vi "Path Type Specialization - Single Converter.vi"(11 "error in":errorcluster) -> (4 "type specialization for path":T1(array[cluster]), 15 "error out":errorcluster)   [LabVIEW 2021, in "Converter.lvlib"]
uses:
  Converter.lvlib
  <vilib>/Utility/traverseref.llb/TRef TravTarget.ctl
  <vilib>/Utility/traverseref.llb/VI Scripting - Traverse.lvlib
  Path Functions/Path Functions.lvlib
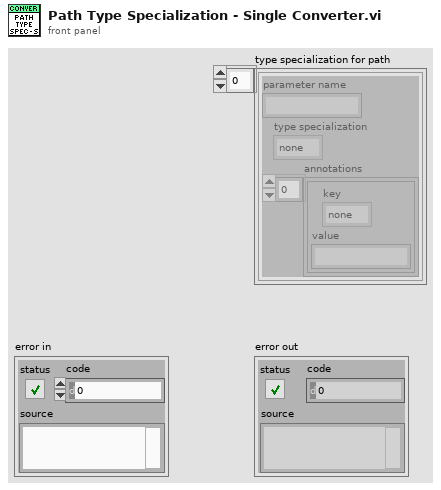
[diagram p1: front panel]
types:
  T1 = cluster{"parameter name":string, "type specialization":enum16{"none", "pin", "path", "enum"}, "annotations":cluster{"key":enum16{"none", "pin.instrument_type", "enum.values"}, "value":string}[]}[]
  T2 = typedef "TRef TravTarget.ctl" = enum16{"FP", "BD", "Other"}
  T3 = cluster{"parameter name":string, "type specialization":enum16{"none", "pin", "path", "enum"}, "annotations":cluster{"key":enum16{"none", "pin.instrument_type", "enum.values"}, "value":string}[]}
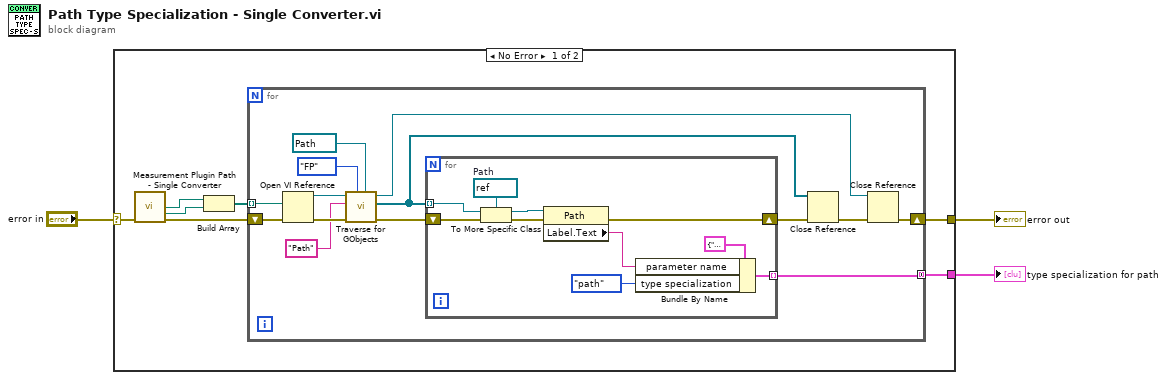
[diagram p0: block diagram]
diagram:
  n1 = case shown="No Error" "error in" {
    selector: "error in" -> [w10 w35]
    tunnel: [w5 w35] -> w2
    tunnel: [w4 _] -> w1
    frame No Error {
      n2 = call "Measurement Plugin Path - Single Converter.vi"("error in"=w10) -> ("result control"=w8:path, "input controls"=w7:path, "error out"=w9:errorcluster)  [unwired: 2 in, 10 out]
      n3 = Build Array(w8, w7) -> (w6:path[])
      n4 = for {
        tunnel: w6 -> [w12] mode=indexing
        shift-right: [w14] -> w5
        shift-left: w9 -> [w23]
        tunnel: [w18] -> w4 mode=concatenating
        n5 = Open VI Reference(vi path=w12, error in (no error)=w23) -> (vi reference=w22:refnum<vi>, error out=w24:errorcluster)  [unwired: 4 in]
        n6 = call <vilib>:"Traverse for GObjects.vi"("Other Refnum"=refnum<vi> refnum, "Traverse Target"=TRef_TravTarget."FP", "error in (no error)"=w24, "Class Name"="Path", "VI Refnum"=w22) -> ("error out"=w19:errorcluster, "References"=w16:refnum<vi>[], "dup VI Refnum"=w15:refnum<vi>)  [unwired: 3 in, 1 out]
        n7 = for {
          shift-right: [w28] -> w17
          shift-left: w19 -> [w34]
          tunnel: w16 -> [w33] mode=indexing
          tunnel: [w27] -> w18 mode=indexing
          w25 = refnum<vi> refnum  # Path
          n8 = To More Specific Class(target class=w25, reference=w33, error in=w34) -> (specific class reference=w31:refnum<vi>, error out=w32:errorcluster)
          n9 = property class="Path"(reference=w31, error in=w32) -> (error out=w28:errorcluster, "Label.Text"=w29:string)  [unwired: 1 out]
          n10 = Bundle By Name(cluster=T3 {"parameter name"="", "type specialization"=enum."none", "annotations"=[]} ("Type Specialization"), "parameter name"=w29, "type specialization"=enum16{"none", "pin", "path", "enum"}."path") -> (w27:T3)
        }
        n11 = Close Reference(reference=w16, error in (no error)=w17) -> (error out=w13:errorcluster)
        n12 = Close Reference(reference=w15, error in (no error)=w13) -> (error out=w14:errorcluster)
      }
    }
    frame Error {
    }
  }
  "error out" <- w2
  "type specialization for path" <- w1
